vi "getReasonText.vi"(10 "Reason":T1 items=["nominal"=0, "unspecified"=1, "left memory"=2, "timed out"=56, "disconnected by peer"=66], 11 "Connection":refnum<class "Connection.lvclass">) -> (2 "Reason message":string)   [LabVIEW 2013, in "MQTT_Connection.lvlib" / "Connection.lvclass"]
uses:
  Connection.lvclass
  reason -- ring.ctl
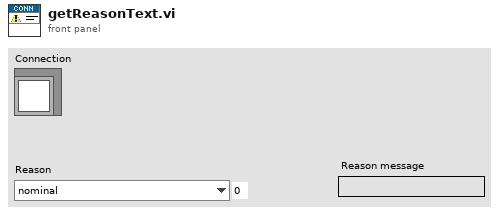
[diagram p1: front panel]
types:
  T1 = typedef "MQTT_Connection.lvlib/Connection.lvclass/reason -- ring.ctl" = u16
  T2 = typedef "LVStringsAndValuesArrayTypeDef_U16.ctl" = cluster{"String":string, "Value":u16}[]
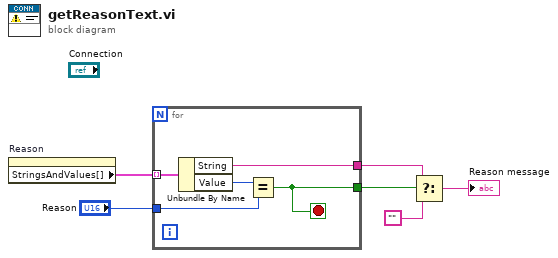
[diagram p0: block diagram]
diagram:
  n1 = property on="Reason" class="Ring (strict)"() -> ("StringsAndValues[]"=w6:T2)  [unwired: 2 in, 2 out]
  n2 = for {
    tunnel: w6 -> [w11] mode=indexing
    tunnel: "Reason" -> [w9]
    tunnel: [w8] -> w4
    tunnel: [w7] -> w3
    stop <- w8 stop-if-true
    n3 = Unbundle By Name(w11) -> ("String"=w7:string, "Value"=w10:u16)
    n4 = Equal?(x=w10, y=w9) -> (x = y?=w8:bool)
  }
  n5 = Select(t=w3, s=w4, f="") -> (s? t:f=→"Reason message":string)
